vi "Remove Ignored Externals.vi"(11 "Externals in":string[](array[string])) -> (3 "Externals out":string[](array[string]))   [LabVIEW 2019, in "Project.Dependencies Finder.lvlib"]
uses:
  Project.Dependencies Finder.lvlib
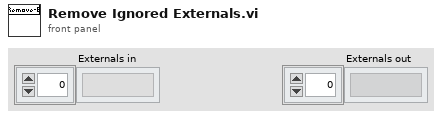
[diagram p1: front panel]
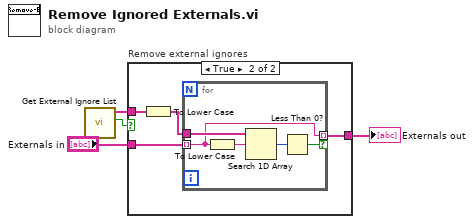
[diagram p0: block diagram]
diagram:
  n1 = call "Get External Ignore List.vi"() -> ("Success?"=w1:bool, "Lower case external ignores"=w3:string[])  [unwired: 10 in]
  n2 = case "Remove external ignores" shown="True" w1 {
    tunnel: "Externals in" -> [w5 w9]
    tunnel: [w5 w7] -> w4
    tunnel: w3 -> [_ w8]
    frame False {
    }
    frame True {
      n3 = To Lower Case(string=w8) -> (all lower case string=w6:string[])
      n4 = for {
        tunnel: w9 -> [w12] mode=indexing
        tunnel: w6 -> [w14]
        tunnel: [w12] -> w7 mode=indexing if=w11
        n5 = To Lower Case(string=w12) -> (all lower case string=w10:string)
        n6 = Search 1D Array(1D array=w14, element=w10) -> (index of element=w13:i32)  [unwired: 1 in]
        n7 = Less Than 0?(x=w13) -> (x < 0?=w11:bool)
      }
    }
  }
  "Externals out" <- w4
